vi "settingsSuffixPath.vi"(2 "settings suffix (_settings)":string="_settings", 3 "path in":path) -> (0 "path out":path)   [LabVIEW 2015]
doc: "Appends to a path the string given as input.\nBy default, appends '_settings'.\nExtension of new path is .txt"
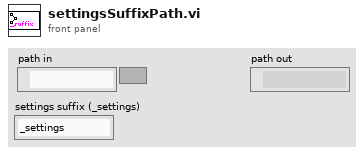
[diagram p1: front panel]
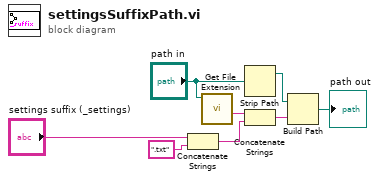
[diagram p0: block diagram]
diagram:
  n1 = Concatenate Strings("settings suffix (_settings)", ".txt" ("string")) -> (w2:string)
  n2 = call <vilib>:"Get File Extension.vi"("file"="path in") -> ("filename without extension"=w6:string)  [unwired: 6 in, 4 out]
  n3 = Strip Path(path="path in") -> (stripped path=w5:path)  [unwired: 1 out]
  n4 = Concatenate Strings(w6, w2) -> (w7:string)
  n5 = Build Path(base path=w5, name or relative path=w7) -> (appended path=→"path out":path)
